vi "SetInitializeController.vi"(8 "error in":errorcluster, 11 "VISA resource name":refnum<visa-resource-name>) -> (0 "error out":errorcluster, 3 "VISA resource name out":refnum<visa-resource-name>)   [LabVIEW 2023, in "Thermotron 8800.lvlib"]
doc: "INIT\nCommand name: Initialize controller\nCommand type: Control\nDescription: This command initializes the 8800.\nSyntax: INIT\nData type: No data\nNOTE: Wait at least one minute after sending this command before sending any other\ncommands."
uses:
  Thermotron 8800.lvlib
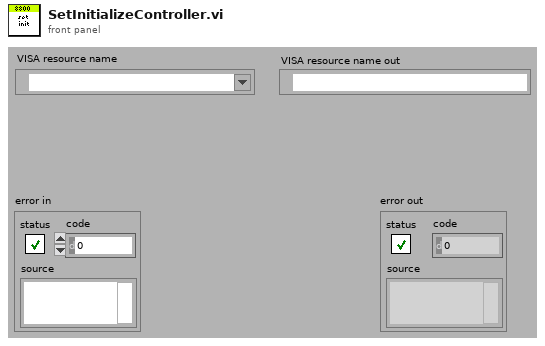
[diagram p1: front panel]
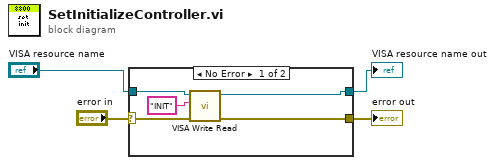
[diagram p0: block diagram]
diagram:
  n1 = case shown="No Error" "error in" {
    selector: "error in" -> [w9 w11]
    tunnel: [w7 w11] -> w1
    tunnel: [w8 w10] -> w2
    tunnel: "VISA resource name" -> [w6 w10]
    frame No Error {
      n2 = call "VISA Write Read.vi"("error in (no error)"=w9, "8800 Command"="INIT", "VISA Refnum in"=w6) -> ("error out"=w7:errorcluster, "VISA Refnum out"=w8:refnum<visa-resource-name>)  [unwired: 6 in, 1 out]
    }
    frame Error {
      # "execute no code if incoming error"
    }
  }
  "VISA resource name out" <- w2
  "error out" <- w1
